vi "WPI_CameraSet Image Size.vi"(8 "error in (no error)":errorcluster, 9 "Size W,H (pix)":cluster{i32, i32}, 10 "Image Size":T2=enum."320x240", 11 "CameraDevRef":T1={"Camera Address"="192.168.0.90", "CameraStatus"={"status"=FALSE, "code"=0, "source"=""}}) -> (0 "error out":errorcluster, 3 "CameraDevRef Out":T1)   [LabVIEW 2017]
doc: "Specifies the size of the image you want the camera to capture. Most cameras support the standard sizes, and many support custom sizes as well.\n\nThis software is licensed. Open the labview\\readme\\WPI Robotics Library Open Source License.txt file for more information."
uses:
  <vilib>/Rock Robotics/WPI/Camera/WPI_CameraImageSize.ctl
  <vilib>/Rock Robotics/WPI/Camera/WPI_CameraDevRef.ctl
  <vilib>/Rock Robotics/WPI/Camera/WPI_CameraSettings Operations.ctl
  <vilib>/vision/driver/NI_Vision_Acquisition_Software.lvlib
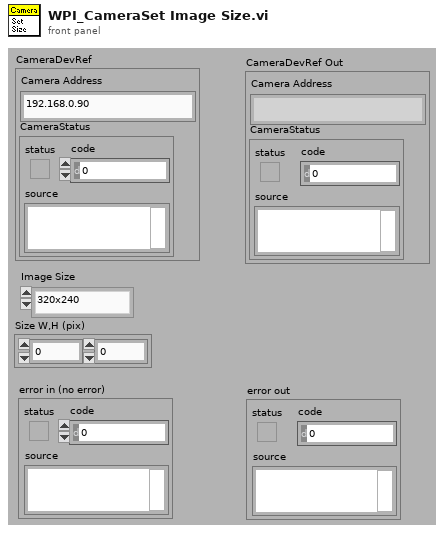
[diagram p1: front panel]
types:
  T1 = typedef "WPI_CameraDevRef.ctl" = cluster{"Camera Address":string, "CameraStatus":errorcluster}
  T2 = typedef "WPI_CameraImageSize.ctl" = enum16{"640x480", "320x240", "160x120", "Custom"}
  T3 = typedef "WPI_CameraSettings Operations.ctl" = enum16{"Udate FPS", "Update Compression", "Update Size", "Update White Balance", "Update Brightness", "Update Sharpness", "Update Exposure", "Update Exposure Value", "Update Color Level", "Update Exp Priority", "Update Color Enable", "Update JPG", "Update MJPG", "Read and Clear", "Read", "Init"}
  T4 = typedef "WPI_CameraSettings Control.ctl" = cluster{"FPS":i32, "Compression":i32, "Size":i32, "White Balance":i32, "Brightness":i32, "Sharpness":i32, "Exposure":i32, "Color Level":i32, "Exposure Priority":i32, "Color Enable":i32, "JPG Loop":i32, "MJPG Loop":i32, "Exposure Value":i32}
  T5 = cluster{"Video Mode":u32, "Video Mode Name":string}[]
  T6 = typedef "IMAQdx.ctl" = refnum<k21>
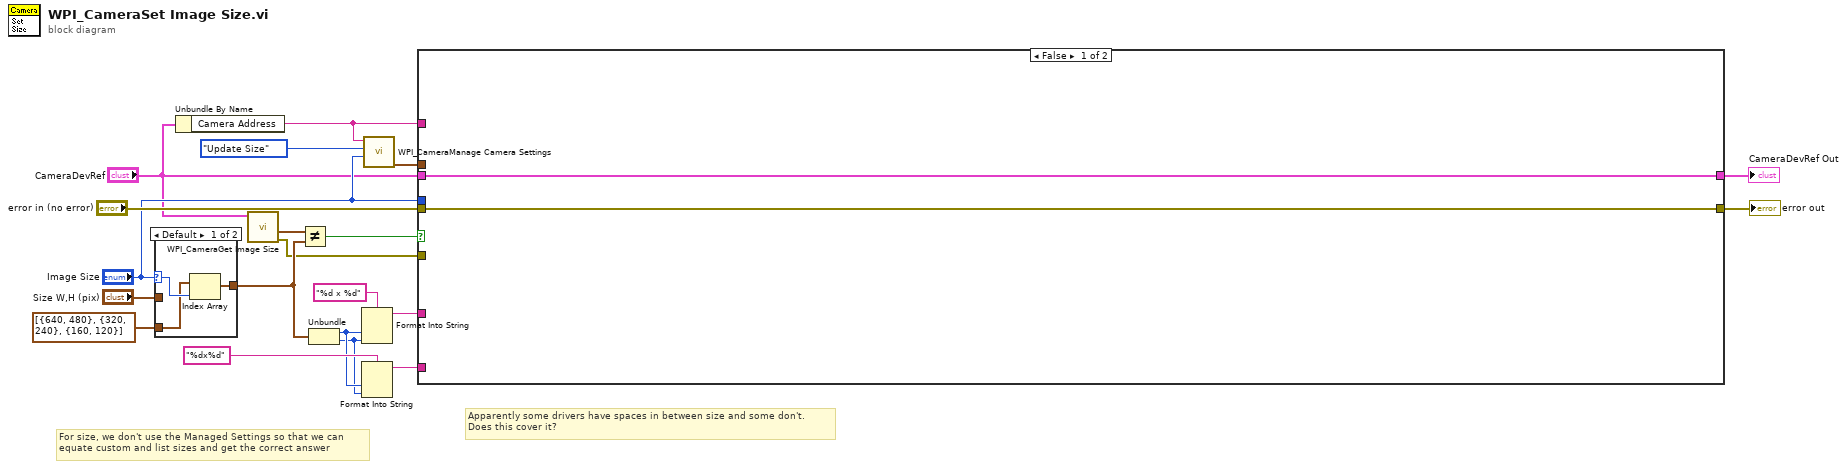
[diagram p0: block diagram]
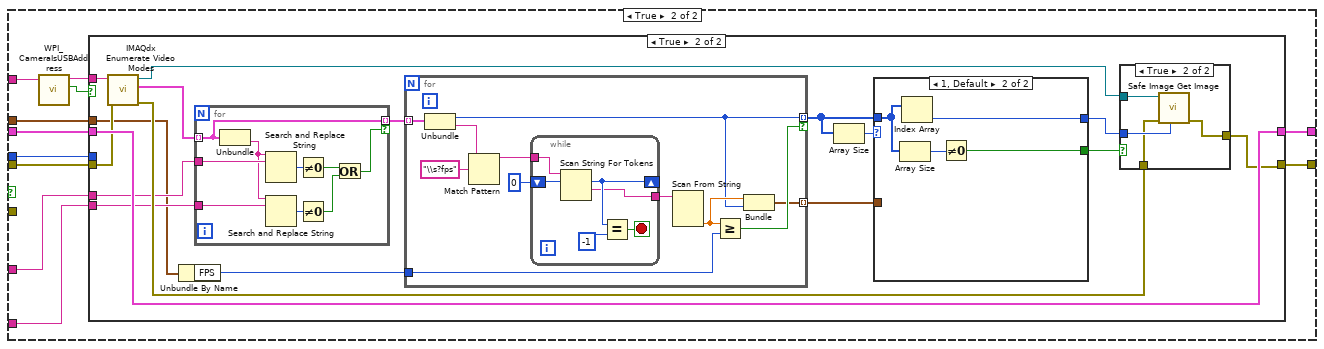
[diagram p3: hidden frame]
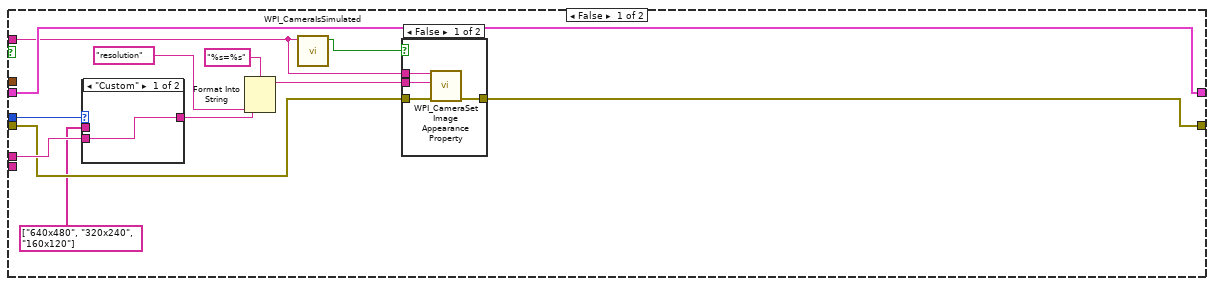
[diagram p4: hidden frame]
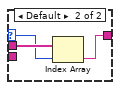
[diagram p6: hidden frame]
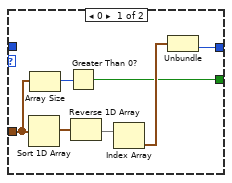
[diagram p7: hidden frame]
diagram:
  # "For size, we don't use the Managed Settings so that we can\nequate custom and list sizes and get the correct answer"
  # "Apparently some drivers have spaces in between size and some don't.\nDoes this cover it?"
  n1 = case shown="Default" "Image Size" {
    selector: "Image Size" -> [w23 _]
    tunnel: "Size W,H (pix)" -> [_ w24]
    tunnel: [w22 w24] -> w2
    tunnel: cluster{i32, i32}[] [{640, 480}, {320, 240}, {160, 120}] -> [w21 _]
    frame Default {
      n2 = Index Array(array=w21, index=w23) -> (element=w22:cluster{i32, i32})
    }
    frame "Custom" {
    }
  }
  n3 = Unbundle By Name("CameraDevRef") -> ("Camera Address"=w16:string)
  n4 = call <vilib>:"WPI_CameraGet Image Size.vi"("CameraDevRef"="CameraDevRef") -> ("error out"=w1:errorcluster, "Size W,H (pix)"=w5:cluster{i32, i32})  [unwired: 7 in, 2 out]
  n5 = Not Equal?(x=w5, y=w2) -> (x != y?=w3:bool)
  n6 = Unbundle(w2) -> (w9:i32, w8:i32)
  n7 = Format Into String(format string="%d x %d" ("Property Name"), w9, w8) -> (resulting string=w11:string)  [unwired: 2 in, 1 out]
  n8 = Format Into String(format string="%dx%d" ("Property Name"), w9, w8) -> (resulting string=w7:string)  [unwired: 2 in, 1 out]
  n9 = call <vilib>:"WPI_CameraManage Camera Settings.vi"("Value"="Image Size", "Operation"=WPI_CameraSettings_Operations."Update Size", "Camera IP"=w16) -> ("Values"=w6:T4)  [unwired: 7 in, 1 out]
  n10 = case shown="False" w3 {
    tunnel: "CameraDevRef" -> [w26 w37]
    tunnel: "Image Size" -> [_ w36]
    tunnel: [w26 w35] -> w20
    tunnel: [w25 w34] -> w19
    tunnel: "error in (no error)" -> [w25 w33]
    tunnel: w16 -> [_ w32]
    tunnel: w11 -> [_ w29]
    tunnel: w7 -> [_ w28]
    tunnel: w6 -> [_ w27]
    tunnel: w1 -> [_ _]
    frame False {
    }
    frame True {
      n11 = call <vilib>:"WPI_CameraIsUSBAddress.vi"("Camera Address In"=w32) -> ("USB?"=w30:bool, "Camera Address Out"=w31:string)  [unwired: 8 in, 1 out]
      n12 = case shown="True" w30 {
        tunnel: w37 -> [w49 w74]
        tunnel: w36 -> [w45 _]
        tunnel: [w49 w74] -> w35
        tunnel: [w42 w73] -> w34
        tunnel: w33 -> [w43 w72]
        tunnel: w31 -> [w39 w68]
        tunnel: w29 -> [w44 w66]
        tunnel: w28 -> [_ w65]
        tunnel: w27 -> [_ w64]
        frame False {
          n13 = case shown="\"Custom\"" w45 {
            selector: w45 -> [_ w56]
            tunnel: string[] ["640x480", "320x240", "160x120"] -> [_ w58]
            tunnel: [w55 w57] -> w47
            tunnel: w44 -> [w55 _]
            frame "Custom" {
            }
            frame Default {
              n14 = Index Array(array=w58, index=w56) -> (element=w57:string)
            }
          }
          n15 = Format Into String(format string="%s=%s", "resolution" ("Property Name"), w47) -> (resulting string=w46:string)  [unwired: 2 in, 1 out]
          n16 = call <vilib>:"WPI_CameraIsSimulated.vi"("Camera Address"=w39) -> ("Simulated"=w40:bool)  [unwired: 10 in]
          n17 = case shown="False" w40 {
            tunnel: w39 -> [w53 _]
            tunnel: w46 -> [w52 _]
            tunnel: w43 -> [w51 w54]
            tunnel: [w50 w54] -> w42
            frame False {
              n18 = call <vilib>:"WPI_CameraSet Image Appearance Property.vi"("error in"=w51, "Prop String"=w52, "address"=w53) -> ("error out"=w50:errorcluster)  [unwired: 1 in, 7 out]
            }
            frame True {
            }
          }
        }
        frame True {
          n19 = call <vilib>:"IMAQdx Enumerate Video Modes.vi"("error in"=w72, "Session In"=w68) -> ("error out"=w71:errorcluster, "Video Modes"=w75:T5, "Session Out"=w67:T6)  [unwired: 6 in, 1 out]
          n20 = Unbundle By Name(w64) -> ("FPS"=w62:i32)
          n21 = for {
            tunnel: w75 -> [w109] mode=indexing
            tunnel: [w109] -> w63 mode=indexing if=w110
            tunnel: w66 -> [w117]
            tunnel: w65 -> [w112]
            n22 = Unbundle(w109) -> ("Video Mode Name"=w111:string)  [unwired: 1 out]
            n23 = Search and Replace String(input string=w111, search string=w117) -> (number of replacements=w116:i32)  [unwired: 6 in, 3 out]
            n24 = Search and Replace String(input string=w111, search string=w112) -> (number of replacements=w114:i32)  [unwired: 6 in, 3 out]
            n25 = Not Equal To 0?(x=w116) -> (x != 0?=w115:bool)
            n26 = Not Equal To 0?(x=w114) -> (x != 0?=w113:bool)
            n27 = Or(x=w115, y=w113) -> (x .or. y?=w110:bool)
          }
          n28 = for {
            tunnel: w63 -> [w97] mode=indexing
            tunnel: [w91] -> w60 mode=indexing if=w93
            tunnel: w62 -> [w94]
            tunnel: [w90] -> w59 mode=indexing
            n29 = Unbundle(w97) -> ("Video Mode"=w91:u32, "Video Mode Name"=w89:string)
            n30 = Match Pattern(string=w89, regular expression="\\s?fps") -> (before substring=w88:string)  [unwired: 1 in, 3 out]
            n31 = while {
              shift-right: [w99] -> _
              shift-left: 0 ("offset past token") -> [w103]
              tunnel: w88 -> [w102]
              tunnel: [w98] -> w95
              stop <- w100 stop-if-true
              n32 = Scan String For Tokens(8:w103, 9:w102) -> (1:w98:string, 2:w99:i32)  [unwired: 4 in, 2 out]
              n33 = Equal?(x=w99, y=-1 ("offset past token")) -> (x = y?=w100:bool)
            }
            n34 = Scan From String(input string=w95) -> (output 1=w92:dbl)  [unwired: 4 in, 3 out]
            n35 = Greater Or Equal?(x=w92, y=w94) -> (x >= y?=w93:bool)
            n36 = Bundle(w92, "Video Mode"=w91) -> (w90:cluster{dbl, "Video Mode":u32})  [unwired: 1 in]
          }
          n37 = Array Size(array=w60) -> (size(s)=w61:i32)
          n38 = case shown="1, Default" w61 {
            tunnel: [w76 w86] -> w70
            tunnel: [w79 w84] -> w69
            tunnel: w60 -> [_ w83]
            tunnel: w59 -> [w78 _]
            frame 0 {
              n39 = Sort 1D Array(array=w78) -> (sorted array=w82:cluster{dbl, "Video Mode":u32}[])
              n40 = Array Size(array=w78) -> (size(s)=w77:i32)
              n41 = Greater Than 0?(x=w77) -> (x > 0?=w76:bool)
              n42 = Reverse 1D Array(array=w82) -> (reversed array=w81:cluster{dbl, "Video Mode":u32}[])
              n43 = Index Array(array=w81) -> (element=w80:cluster{dbl, "Video Mode":u32})  [unwired: 1 in]
              n44 = Unbundle(w80) -> ("Video Mode"=w79:u32)  [unwired: 1 out]
            }
            frame 1, Default {
              n45 = Array Size(array=w83) -> (size(s)=w85:i32)
              n46 = Index Array(array=w83) -> (element=w84:u32)  [unwired: 1 in]
              n47 = Not Equal To 0?(x=w85) -> (x != 0?=w86:bool)
            }
          }
          n48 = case shown="True" w70 {
            tunnel: w69 -> [_ w107]
            tunnel: w67 -> [_ w105]
            tunnel: w71 -> [w104 w106]
            tunnel: [w104 w108] -> w73
            frame False {
            }
            frame True {
              n49 = call <vilib>:"Safe Image Get Image.vi"("Video Mode"=w107, "error in"=w106, "Session In"=w105) -> ("error out"=w108:errorcluster)  [unwired: 5 in, 3 out]
            }
          }
        }
      }
    }
  }
  "CameraDevRef Out" <- w20
  "error out" <- w19
